vi "输出控制.vi"() -> (3 "输出控制输出":T1)   [LabVIEW 2017]
panel:
  in  "选项卡控件":enum32{"选项卡 1", "选项卡 2"}(tab)
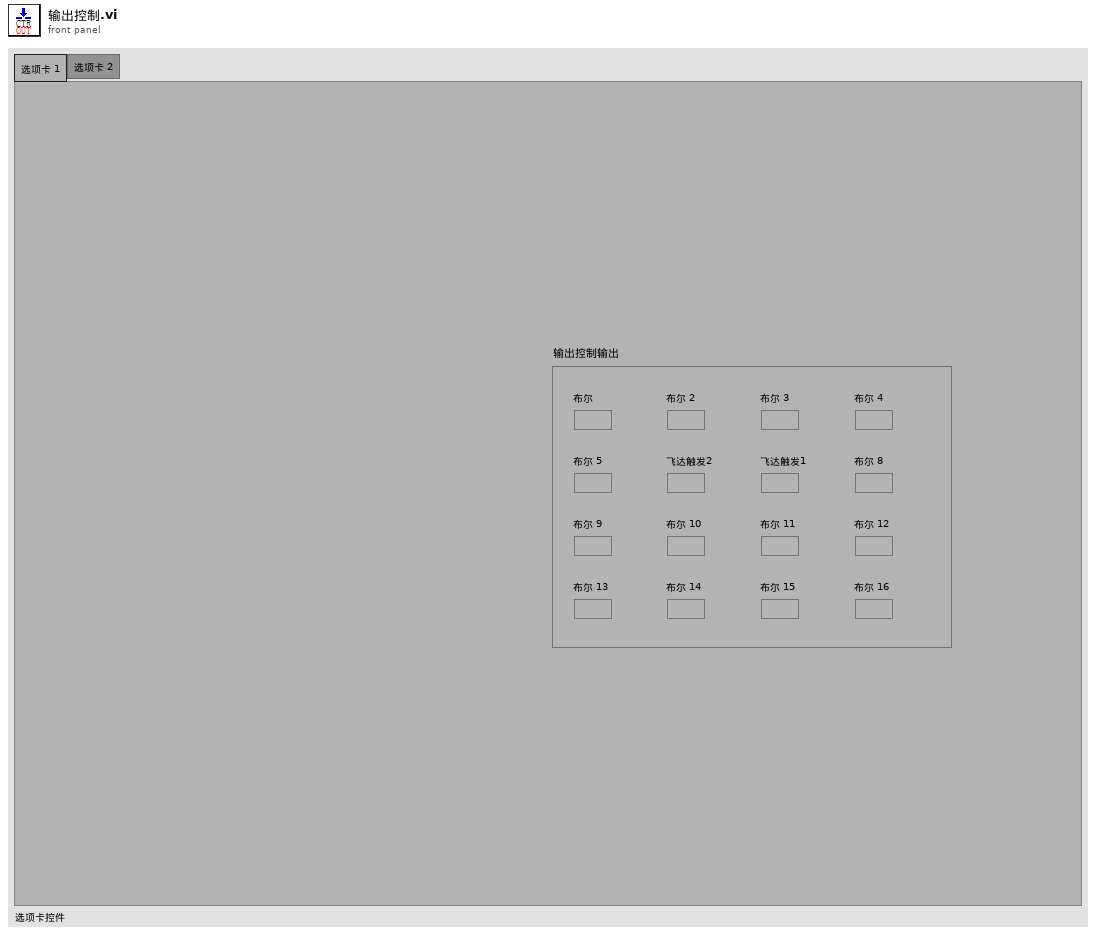
[diagram p1: front panel]
types:
  T1 = typedef "output控件.ctl" = cluster{"布尔":bool, "布尔 2":bool, "布尔 3":bool, "布尔 4":bool, "布尔 5":bool, "飞达触发2":bool, "飞达触发1":bool, "布尔 8":bool, "布尔 9":bool, "布尔 10":bool, "布尔 11":bool, "布尔 12":bool, "布尔 13":bool, "布尔 14":bool, "布尔 15":bool, "布尔 16":bool}
  T2 = typedef "MX操作选项.ctl" = enum16{"MX Initial ", "MX Close", "X&Y&M Read", "X&Y&M Write", "D Read", "D Write", "Many component Read", "Many component Write", "Load Function Global"}
  T3 = typedef "Component Assemble Input.ctl" = cluster{"Component Name":string, "Component State":bool, "D Value":i32}
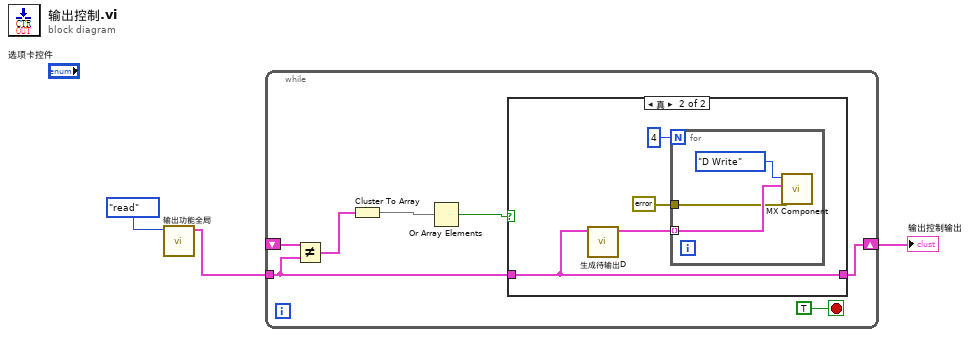
[diagram p0: block diagram]
diagram:
  n1 = call "输出功能全局.vi"("选项"=enum16{"initialize", "read", "write"}."read") -> ("输出"=w1:T1)  [unwired: 10 in]
  n2 = while {
    shift-right: [w9] -> w3
    shift-left: _ -> [w8]
    tunnel: w1 -> [w7]
    stop <- TRUE stop-if-true
    n3 = Not Equal?(x=w8, y=w7) -> (x != y?=w4:T1)
    n4 = Cluster To Array(cluster=w4) -> (array=w6:bool[])
    n5 = Or Array Elements(Boolean array=w6) -> (logical OR=w5:bool)
    n6 = case shown="真" w5 {
      tunnel: w7 -> [w11 w13]
      tunnel: [w11 w13] -> w9
      frame False {
      }
      frame True {
        n7 = call "生成待输出D.vi"("输出"=w13) -> ("待输出操作"=w12:T3[])  [unwired: 10 in]
        n8 = for {
          N: 4 -> [_]
          tunnel: w12 -> [w17] mode=indexing
          tunnel: errorcluster {"status"=FALSE, "code"=0, "source"=""} ("错误输入") -> [w16]
          n9 = call "MX Component.vi"("错误输入"=w16, "Component Assemble Input"=w17, "MX操作选项"=MX操作选项."D Write") -> ()  [unwired: 6 in, 3 out]
        }
      }
    }
  }
  "输出控制输出" <- w3
